vi "Get Project Path.vi"(11 "CD Build Tools in":refnum<class "Project Build Tools.lvclass">) -> (2 "Project Path":path, 3 "CD Build Tools out":refnum<class "Project Build Tools.lvclass">)   [LabVIEW 2019, in "Project Build Tools.lvclass"]
uses:
  Project Build Tools.lvclass
  Project Build Tools.lvclass/Project Build Tools.ctl
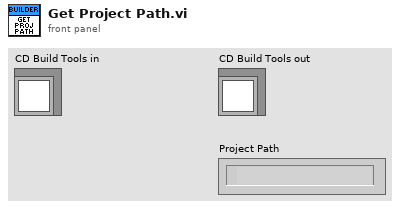
[diagram p1: front panel]
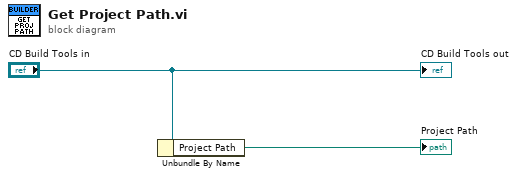
[diagram p0: block diagram]
diagram:
  n1 = Unbundle By Name("CD Build Tools in") -> ("Project Path"=→"Project Path":path)
  "CD Build Tools out" <- "CD Build Tools in"
